vi "ex4 .vi"() -> ()   [LabVIEW 2019]
uses:
  <vilib>/myRIO/Instrument Drivers/Onboard IO/I2C/typedefs/I2C User Configuration.ctl
  <vilib>/myRIO/Instrument Drivers/Onboard IO/I2C/typedefs/I2C Transfer Rate.ctl
  <vilib>/myRIO/Instrument Drivers/Onboard IO/I2C/typedefs/I2C Reference.ctl
  <vilib>/myRIO/Common/Instrument Driver Framework/Utilities/typedefs/myRIO Generic Hardware Reference.ctl
  <vilib>/myRIO/Common/Instrument Driver Framework/Utilities/typedefs/Hardware Version Enum.ctl
  <vilib>/myRIO/Common/Instrument Driver Framework/Utilities/typedefs/myRIO v1.0 Reference.ctl
  <vilib>/myRIO/Common/Instrument Driver Framework/Utilities/typedefs/Generic FPGA Reference.ctl
  <vilib>/myRIO/Common/Instrument Driver Framework/myRIO v1.0/I2C/typedefs/I2C Channels Enum.ctl
  <vilib>/myRIO/Instrument Drivers/Onboard IO/I2C/typedefs/I2C Configuration.ctl
  <vilib>/userDefined/High Color/nirio_resource_hc.ctl
  <vilib>/myRIO/Common/Instrument Driver Framework/Utilities/vis/Is FPGA Ref Available.vi
  <vilib>/myRIO/Common/Instrument Driver Framework/myRIO v1.0/I2C/vis/myRIO v1.1 Open I2C.vi
  <vilib>/myRIO/Instrument Drivers/Onboard IO/I2C/vis/Configure.vi
  <vilib>/myRIO/Instrument Drivers/Onboard IO/I2C/vis/Write.vi
  <vilib>/myRIO/Instrument Drivers/Onboard IO/I2C/vis/Read.vi
  <vilib>/myRIO/Common/Instrument Driver Framework/Utilities/vis/Validate Channels.vi
  <vilib>/myRIO/Common/Instrument Driver Framework/myRIO v1.0/I2C/vis/myRIO v1.0 Reserve I2C.vi
  <vilib>/myRIO/Common/Instrument Driver Framework/myRIO v1.0/I2C/vis/myRIO v1.0 Build MUX Configuration I2C.vi
  <vilib>/myRIO/Common/Instrument Driver Framework/myRIO v1.0/Resource Manager/vis/myRIO v1.0 Reserve Channel List.vi
  <vilib>/myRIO/Common/Instrument Driver Framework/myRIO v1.0/Resource Manager/vis/myRIO v1.0 Create Configuration List.vi
  <vilib>/myRIO/Common/Instrument Driver Framework/myRIO v1.0/Resource Manager/vis/myRIO v1.0 Reserve Channel.vi
  <vilib>/myRIO/Common/Instrument Driver Framework/myRIO v1.0/Resource Manager/vis/myRIO v1.0 Unreserve Channel.vi
  <vilib>/myRIO/Common/Instrument Driver Framework/myRIO v1.0/Resource Manager/vis/myRIO v1.0 Build Mutex Name.vi
  <vilib>/Utility/VariantDataType/GetNumericInfo.vi
  <vilib>/Utility/error.llb/Error Cluster From Error Code.vi
  <vilib>/myRIO/Common/Instrument Driver Framework/myRIO v1.0/myRIO v1.1 Open.vi
  <vilib>/myRIO/Common/Instrument Driver Framework/Utilities/vis/IO Manager.vi
  <vilib>/myRIO/Common/Instrument Driver Framework/Utilities/vis/Configuration Manager.vi
  <vilib>/myRIO/Common/Instrument Driver Framework/myRIO v1.0/Resource Manager/vis/myRIO v1.0 Configure IO.vi
  <vilib>/myRIO/Common/Instrument Driver Framework/myRIO v1.0/myRIO v1.0 Close.vi
  <vilib>/myRIO/Common/Instrument Driver Framework/myRIO v1.0/I2C/vis/myRIO v1.0 Configure I2C.vi
  <vilib>/myRIO/Common/Instrument Driver Framework/myRIO v1.0/I2C/vis/myRIO v1.0 Write I2C.vi
  <vilib>/myRIO/Common/Instrument Driver Framework/myRIO v1.0/I2C/vis/myRIO v1.0 Read I2C.vi
  <vilib>/myRIO/Express VI/Onboard IO/I2C/I2C Express VI.xnode
  <vilib>/myRIO/Instrument Drivers/Onboard IO/I2C/vis/myRIO I2C Open.xnode
  <vilib>/myRIO/Instrument Drivers/Onboard IO/I2C/I2C.lvlib
panel:
  out "Bytes Read magnet Z":u8[](array[numeric])
  out "Bytes Read magnet Y":u8[](array[numeric])
  out "Bytes Read magnet X":u8[](array[numeric])
  out "Bytes Read Z":u8[](array[numeric])
  out "Bytes Read Y":u8[](array[numeric])
  out "Bytes Read X":u8[](array[numeric])
  in  "stop":bool
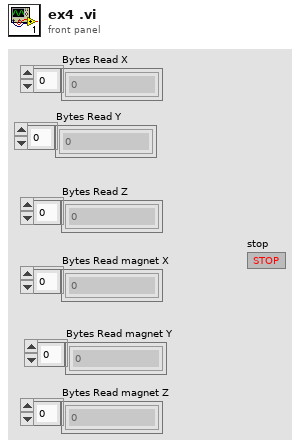
[diagram p1: front panel]
types:
  T1 = typedef "I2C.lvlib/I2C Reference.ctl" = cluster{"myRIO Reference":T2, "I2C Channels Enum":T6, "I2C Configuration":T7}
  T2 = typedef "myRIO Generic Hardware Reference.ctl" = cluster{"myRIO Model":T3, "myRIO Hardware Reference":T4}
  T3 = typedef "Hardware Version Enum.ctl" = enum16{"Unknown", "myRIO-1900", "myRIO-1950", "roboRIO", "NI ELVIS RIO CM", "ELVIS III"}
  T4 = typedef "myRIO v1.0 Reference.ctl" = cluster{"Generic FPGA Reference":T5, "Allow multiple opens":bool}
  T5 = typedef "Generic FPGA Reference.ctl" = refnum<k20>
  T6 = typedef "I2C Channels Enum.ctl" = enum16{"Not Connected", "A/I2C", "B/I2C", "I2C/I2C"}
  T7 = typedef "I2C.lvlib/I2C Configuration.ctl" = cluster{"I2C Transfer Rate":T8}
  T8 = typedef "I2C.lvlib/I2C Transfer Rate.ctl" = enum16{"Standard mode (100 kbps)", "Fast mode (400 kbps)"}
  T9 = typedef "I2C.lvlib/I2C User Configuration.ctl" = cluster{"I2C Transfer Rate":T8}
  T10 = typedef "nirio_resource_hc.ctl" = tag
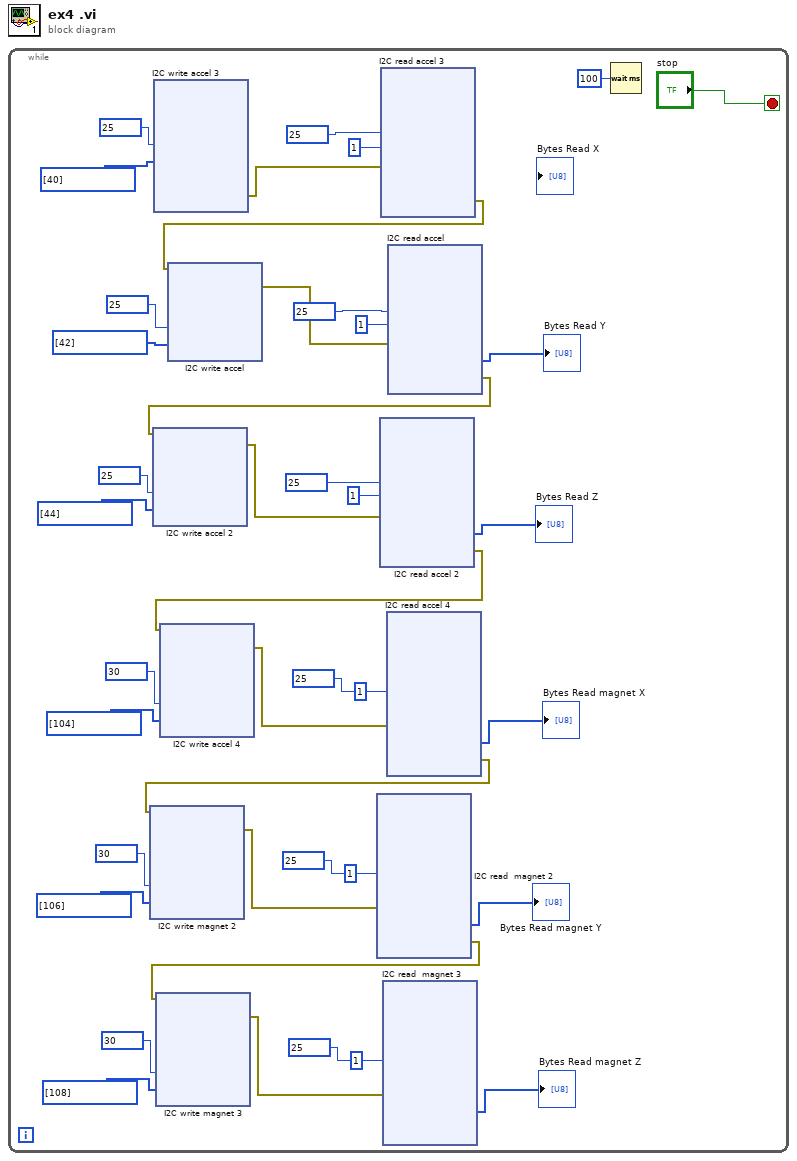
[diagram p0: block diagram]
diagram:
  n1 = while {
    stop <- "stop" stop-if-true
    n2 = xnode "I2C write accel 3"("Slave Address (7-bit)"=u8 25, "Bytes to Write"=u8[] [40]) -> ("error out"=w38:errorcluster)  [unwired: 1 in]
    n3 = xnode "I2C read accel 3"("Slave Address (7-bit)"=u8 25, "Byte Count"=u32 1, "error in (no error)"=w38) -> ("error out"=w7:errorcluster)  [unwired: 1 out]
    n4 = xnode "I2C write accel"("Slave Address (7-bit)"=u8 25, "Bytes to Write"=u8[] [42], "error in (no error)"=w7) -> ("error out"=w37:errorcluster)
    n5 = xnode "I2C read accel"("Slave Address (7-bit)"=u8 25, "Byte Count"=u32 1, "error in (no error)"=w37) -> ("Bytes Read"=→"Bytes Read Y":u8[], "error out"=w6:errorcluster)
    n6 = xnode "I2C write accel 2"("Slave Address (7-bit)"=u8 25, "Bytes to Write"=u8[] [44], "error in (no error)"=w6) -> ("error out"=w26:errorcluster)
    n7 = xnode "I2C read accel 2"("Slave Address (7-bit)"=u8 25, "Byte Count"=u32 1, "error in (no error)"=w26) -> ("Bytes Read"=→"Bytes Read Z":u8[], "error out"=w5:errorcluster)
    n8 = xnode "I2C write accel 4"("Slave Address (7-bit)"=u8 30, "Bytes to Write"=u8[] [104], "error in (no error)"=w5) -> ("error out"=w20:errorcluster)
    n9 = xnode "I2C read accel 4"("Slave Address (7-bit)"=u8 25, "Byte Count"=u32 1, "error in (no error)"=w20) -> ("Bytes Read"=→"Bytes Read magnet X":u8[], "error out"=w4:errorcluster)
    n10 = xnode "I2C write magnet 2"("Slave Address (7-bit)"=u8 30, "Bytes to Write"=u8[] [106], "error in (no error)"=w4) -> ("error out"=w14:errorcluster)
    n11 = xnode "I2C read  magnet 2"("Slave Address (7-bit)"=u8 25, "Byte Count"=u32 1, "error in (no error)"=w14) -> ("Bytes Read"=→"Bytes Read magnet Y":u8[], "error out"=w3:errorcluster)
    n12 = xnode "I2C write magnet 3"("Slave Address (7-bit)"=u8 30, "Bytes to Write"=u8[] [108], "error in (no error)"=w3) -> ("error out"=w8:errorcluster)
    n13 = xnode "I2C read  magnet 3"("Slave Address (7-bit)"=u8 25, "Byte Count"=u32 1, "error in (no error)"=w8) -> ("Bytes Read"=→"Bytes Read magnet Z":u8[])  [unwired: 1 out]
    n14 = Wait (ms)(milliseconds to wait=u32 100) -> ()  [unwired: 1 out]
  }
